vi "Get Parameter Value (array).vi"(10 "Parameter Name":string, 11 "JSON":string) -> (1 "Found":bool, 2 "Parameter Values":string[](array[string]), 3 "Remaining JSON":string)   [LabVIEW 2015, in "NI_JSON Parsing.lvlib"]
uses:
  NI_JSON Parsing.lvlib
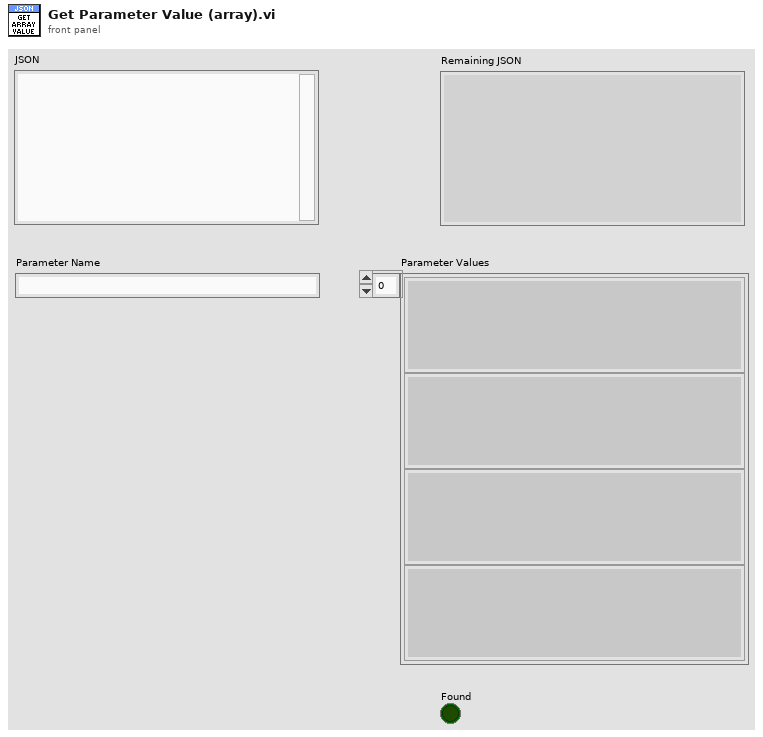
[diagram p1: front panel]
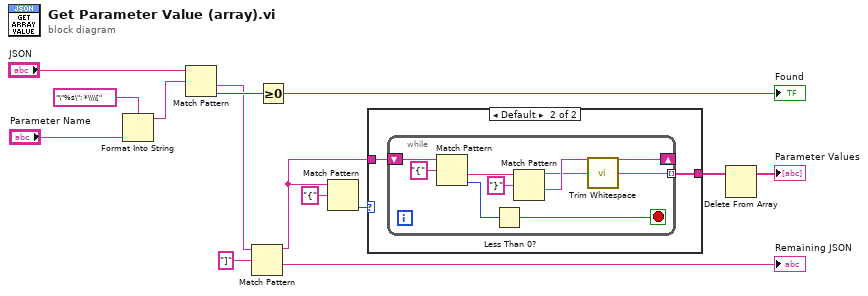
[diagram p0: block diagram]
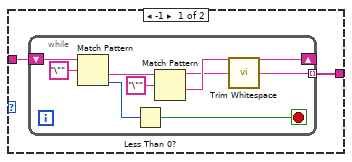
[diagram p2: hidden frame]
diagram:
  n1 = Format Into String(format string="\"%s\": *\\\\[", "Parameter Name") -> (resulting string=w7:string)  [unwired: 2 in, 1 out]
  n2 = Match Pattern(string="JSON", regular expression=w7) -> (after substring=w4:string, offset past match=w6:i32)  [unwired: 1 in, 2 out]
  n3 = Match Pattern(string=w4, regular expression="]") -> (before substring=w3:string, after substring=→"Remaining JSON":string)  [unwired: 1 in, 2 out]
  n4 = Greater Or Equal To 0?(x=w6) -> (x >= 0?=→"Found":bool)
  n5 = Match Pattern(string=w3, regular expression="{") -> (offset past match=w1:i32)  [unwired: 1 in, 3 out]
  n6 = case shown="Default" w1 {
    tunnel: [w16 w27] -> w12
    tunnel: w3 -> [w15 w26]
    frame -1 {
      n7 = while {
        shift-right: [w20] -> _
        shift-left: w15 -> [w25]
        tunnel: [w17] -> w16 mode=indexing
        stop <- w22 stop-if-true
        n8 = Match Pattern(string=w25, regular expression="\"") -> (after substring=w21:string, offset past match=w23:i32)  [unwired: 1 in, 2 out]
        n9 = Less Than 0?(x=w23) -> (x < 0?=w22:bool)
        n10 = Match Pattern(string=w21, regular expression="\"") -> (before substring=w18:string, after substring=w20:string)  [unwired: 1 in, 2 out]
        n11 = call <vilib>:"Trim Whitespace.vi"("string"=w18) -> ("trimmed string"=w17:string)  [unwired: 1 in]
      }
    }
    frame Default {
      n12 = while {
        shift-right: [w31] -> _
        shift-left: w26 -> [w36]
        tunnel: [w28] -> w27 mode=indexing
        stop <- w33 stop-if-true
        n13 = Match Pattern(string=w36, regular expression="{") -> (after substring=w32:string, offset past match=w34:i32)  [unwired: 1 in, 2 out]
        n14 = Less Than 0?(x=w34) -> (x < 0?=w33:bool)
        n15 = Match Pattern(string=w32, regular expression="}") -> (before substring=w29:string, after substring=w31:string)  [unwired: 1 in, 2 out]
        n16 = call <vilib>:"Trim Whitespace.vi"("string"=w29) -> ("trimmed string"=w28:string)  [unwired: 1 in]
      }
    }
  }
  n17 = Delete From Array(array=w12) -> (array with subset deleted=→"Parameter Values":string[])  [unwired: 2 in, 1 out]
